vi "Configure Trace Display.vi"(0 "VISA resource name":refnum<visa-resource-name>, 1 "Channel (1)":i32=1, 3 "Trace (1)":i32=1, 5 "Trace Display (0: Normal Data)":u16(ring) items=["Normal Data", "Data + Memory", "Data - Memory", "Data * Memory", "Data / Memory"], 7 "Display Data (T: Enable)":bool=TRUE, 9 "Display Memory (T: Enable)":bool=TRUE, 11 "error in (no error)":errorcluster) -> (4 "VISA resource name out":refnum<visa-resource-name>, 15 "error out":errorcluster)   [LabVIEW 2011, in "Agilent ENA Series.lvlib"]
doc: "This VI configures display of active trace."
uses:
  Agilent ENA Series.lvlib
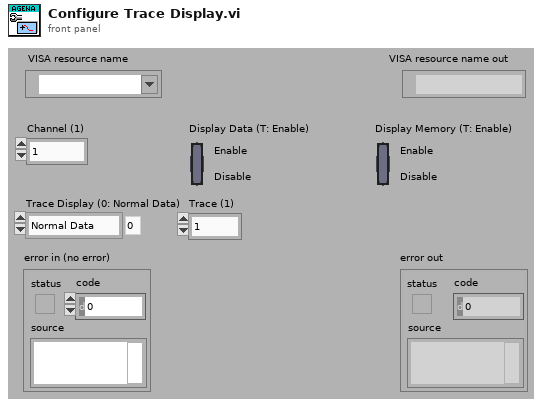
[diagram p1: front panel]
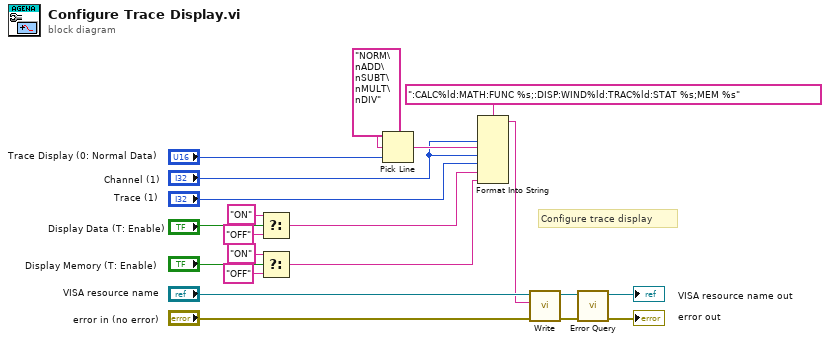
[diagram p0: block diagram]
diagram:
  # "Configure trace display"
  n1 = Select(t="ON", s="Display Data (T: Enable)", f="OFF" ("t")) -> (s? t:f=w7:string)
  n2 = Select(t="ON", s="Display Memory (T: Enable)", f="OFF" ("t")) -> (s? t:f=w6:string)
  n3 = Pick Line(multi-line string="NORM\nADD\nSUBT\nMULT\nDIV", line index="Trace Display (0: Normal Data)") -> (output string=w10:string)  [unwired: 1 in]
  n4 = Format Into String(format string=":CALC%ld:MATH:FUNC %s;:DISP:WIND%ld:TRAC%ld:STAT %s;MEM %s", "Channel (1)", w10, "Channel (1)", "Trace (1)", w7, w6) -> (resulting string=w5:string)  [unwired: 2 in, 1 out]
  n5 = call "Write.vi"("error in (no error)"="error in (no error)", "String ()"=w5, "VISA resource name"="VISA resource name") -> ("error out"=w3:errorcluster, "VISA resource name out"=w4:refnum<visa-resource-name>)  [unwired: 6 in, 1 out]
  n6 = call "Error Query.vi"("error in (no error)"=w3, "VISA resource name"=w4) -> ("error out"=→"error out":errorcluster, "VISA resource name out"=→"VISA resource name out":refnum<visa-resource-name>)  [unwired: 6 in, 2 out]
